vi "Read Value.vi"(8 "error in (no error)":errorcluster, 11 "fixed32 in":refnum<class "bytes.lvclass">) -> (0 "error out":errorcluster, 2 "Value":u8[](array[numeric]), 3 "fixed32 out":refnum<class "bytes.lvclass">)   [LabVIEW 2020, in "Protobuf RAW.lvlib" / "bytes.lvclass"]
uses:
  bytes.lvclass
  bytes.lvclass/bytes.ctl
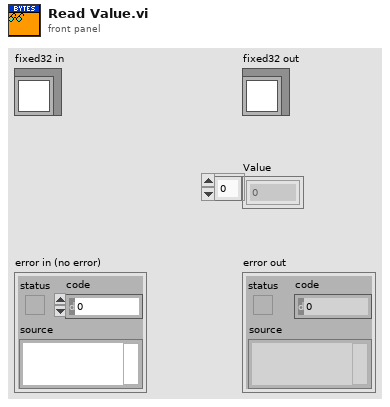
[diagram p1: front panel]
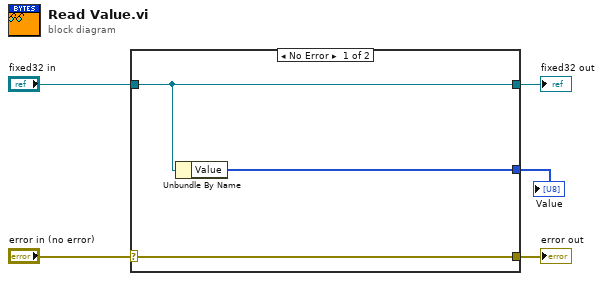
[diagram p0: block diagram]
diagram:
  n1 = case shown="No Error" "error in (no error)" {
    selector: "error in (no error)" -> [w8 w9]
    tunnel: [w8 w9] -> w4
    tunnel: [w7 w10] -> w2
    tunnel: "fixed32 in" -> [w7 w10]
    tunnel: [w6 _] -> w1
    frame No Error {
      n2 = Unbundle By Name(w7) -> ("Value"=w6:u8[])
    }
    frame Error {
    }
  }
  "error out" <- w4
  "fixed32 out" <- w2
  "Value" <- w1
